vi "Global.vi"() -> ()   [LabVIEW 2010, in "XNET Reflective Memory Custom Device.lvlib"]
uses:
  XNET Reflective Memory Custom Device.lvlib
  RT DATA.ctl
  Single Category.ctl
  BeforeAfter.ctl
  <vilib>/NI Veristand/Custom Device API/Data Reference.ctl
  <vilib>/NI Veristand/Custom Device API/Custom Device API.lvlib
panel:
  in  "Master?":string="StartTrig"
  in  "RT DATA":T1={" Inputs"={"Vals"=[], "When"=[], "Data Refs"=[], "Session"="", "NIT Start"=0}, "Outputs"={"Vals"=[], "When"=[], "Data Refs"=[], "Session"="", "NIT Start"=0}, "Internal Iteration"=-2, "Device Error"={"status"=FALSE, "code"=0, "source"=""}} {"Outputs"."Data Refs" format="%.0x"; "Inputs"."Data Refs" format="%.0x"}
  in  "KeySlot":string="KeySlot"
  in  "ColdStart?":string="ColdStart?"
  in  "Database":string="Database"
  in  "Cluster":string="Cluster"
  in  "Channel Page GUID":string="ED3BC212-561D-6BFC-077C-45C4CFB04B45"
  in  "Interface":string="Interface"
  in  "BeforeAfter?":string="BeforeAfter?"
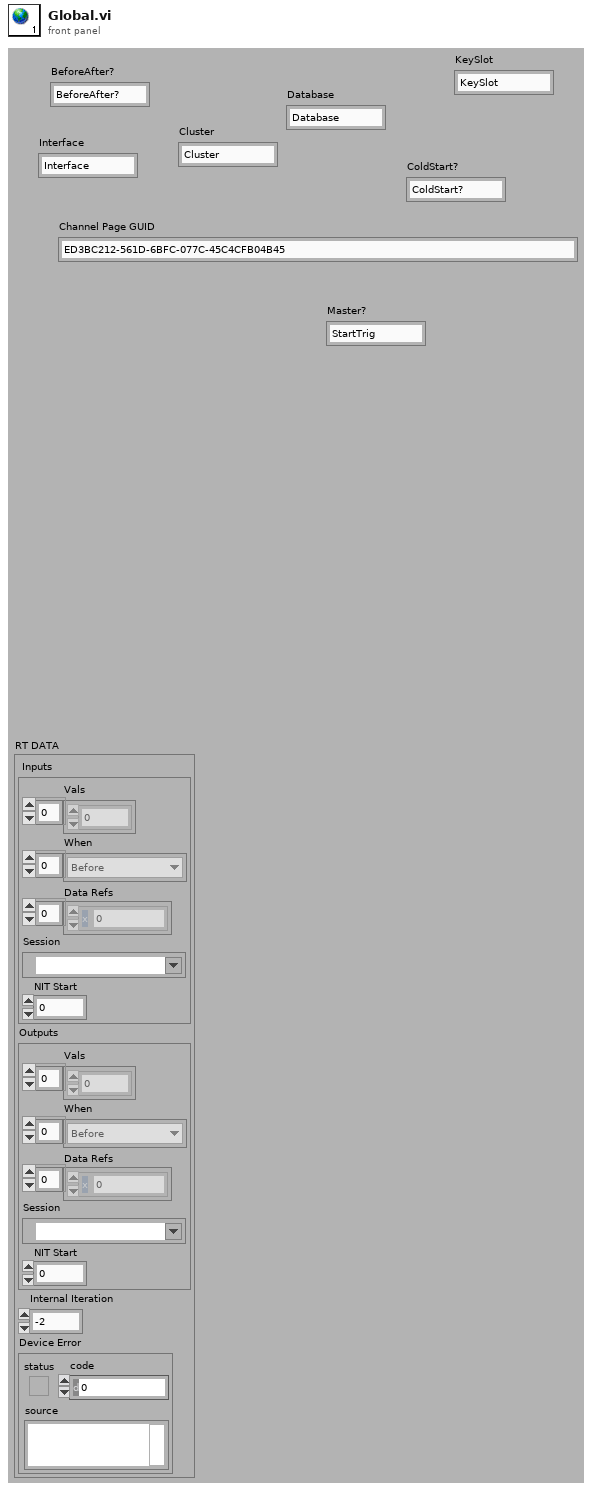
[diagram p1: front panel]
types:
  T1 = typedef "XNET Reflective Memory Custom Device.lvlib/RT DATA.ctl" = cluster{" Inputs":T2, "Outputs":T2, "Internal Iteration":i32, "Device Error":errorcluster}
  T2 = typedef "XNET Reflective Memory Custom Device.lvlib/Single Category.ctl" = cluster{"Vals":dbl[], "When":T3[], "Data Refs":T4[], "Session":refnum<k21>, "NIT Start":u32}
  T3 = typedef "XNET Reflective Memory Custom Device.lvlib/BeforeAfter.ctl" = enum16{"Before", "After"}
  T4 = typedef "Custom Device API.lvlib/Data Reference.ctl" = i32
diagram:
